vi "Get Monitors.vi"(0 "fpga interface in":refnum<k20>, 11 "error in (no error)":errorcluster) -> (4 "fpga interface out":refnum<k20>, 6 "FPGA Temperature (C)":dbl, 8 "Temperature Limit (C)":dbl, 10 "Total Power (W)":dbl, 14 "Power Limit (W)":dbl, 15 "error out":errorcluster)   [LabVIEW 2018, in "GettingStarted_5775_Host.lvlib"]
uses:
  GettingStarted_5775_Host.lvlib
  <instrlib>/FlexRIO/API/Host/v1/NI FlexRIO/API/Get Property Reference - Fpga Small.vi
  <resource>/objmgr/niflexrioapi.rc
  <instrlib>/FlexRIO/API/Host/v1/NI FlexRIO API v1.lvlib
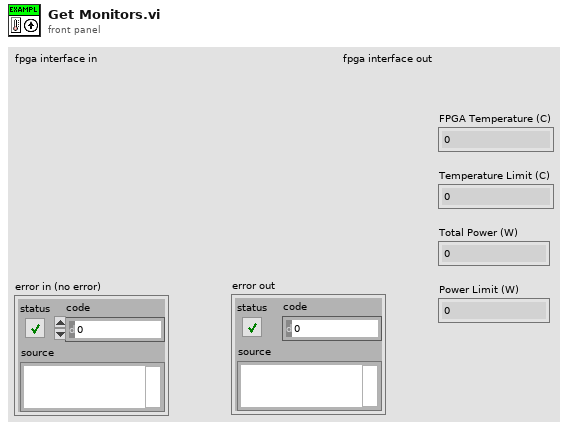
[diagram p1: front panel]
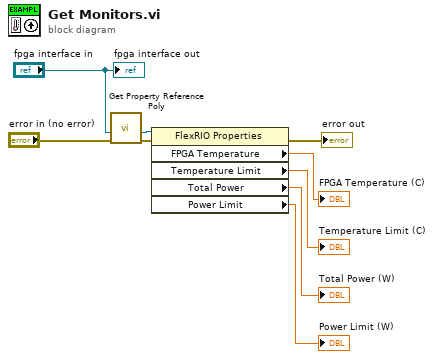
[diagram p0: block diagram]
diagram:
  n1 = call-poly <instrlib>:"Get Property Reference Poly.vi"("error in (no error)"="error in (no error)", "fpga interface in"="fpga interface in") -> ("error out"=w8:errorcluster, "property reference"=w9:refnum<k20>)  [unwired: 4 in, 1 out]
  n2 = property class="FlexRIO Properties"(reference=w9, error in=w8) -> (error out=→"error out":errorcluster, "FPGA Temperature"=→"FPGA Temperature (C)":dbl, "Temperature Limit"=→"Temperature Limit (C)":dbl, "Total Power"=→"Total Power (W)":dbl, "Power Limit"=→"Power Limit (W)":dbl)  [unwired: 1 out]
  "fpga interface out" <- "fpga interface in"
